vi "Get Fix Type.vi"(8 "error in (no error)":errorcluster, 11 "nmea in":refnum<class "nmea.lvclass">) -> (0 "error out":errorcluster, 2 "Fix Type":T1, 3 "nmea out":refnum<class "nmea.lvclass">)   [LabVIEW 2020, in "nmea.lvlib" / "nmea.lvclass"]
uses:
  nmea.lvclass
  Fix Type.ctl
  nmea.lvclass/nmea.ctl
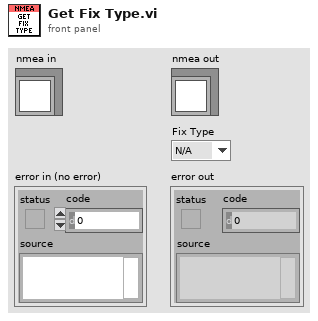
[diagram p1: front panel]
types:
  T1 = typedef "nmea.lvlib/nmea.lvclass/Fix Type.ctl" = enum16{"N/A", "None", "2D", "3D"}
  T2 = typedef "nmea.lvlib/nmea.lvclass/Ref Data.ctl" = cluster{"Latitude":dbl, "Longitude":dbl, "Time":T3, "Status":string, "Speed":dbl, "Course":dbl, "Mag Var":dbl, "Var Dir":string, "Mode":string, "Satellites":T4[], "Next Satellites":T4[], "Active PRNs":i32[], "Fix Type":T1, "DOP":T5, "Fix Mode":T6, "Altitude":dbl, "Geoid":dbl}
  T3 = typedef "LVDateTimeRec.ctl" = cluster{"fractional second":dbl, "second":i32, "minute":i32, "hour":i32, "day of month":i32, "month":i32, "year":i32, "day of week":i32, "day of year":i32, "DST":i32}
  T4 = typedef "nmea.lvlib/nmea.lvclass/Satellite.ctl" = cluster{"PRN":u8, "Channel":u8, "Elevation":u8, "Azimuth":u16, "SNR":u8, "Active":bool}
  T5 = typedef "nmea.lvlib/nmea.lvclass/DOP.ctl" = cluster{"P":dbl, "H":dbl, "V":dbl}
  T6 = typedef "nmea.lvlib/nmea.lvclass/Fix Mode.ctl" = enum16{"Manual", "Auto 2/3D"}
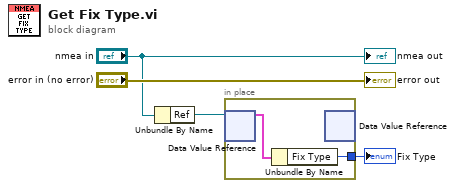
[diagram p0: block diagram]
diagram:
  n1 = Unbundle By Name("nmea in") -> ("Ref"=w3:refnum<data-value>)
  n2 = in-place {
    in-place-border: [w5] -> w1
    n3 = in-place-dvr #1(w3) -> (w6:T2)  [unwired: 1 out]
    n4 = Unbundle By Name(w6) -> ("Fix Type"=w5:T1)
    n5 = in-place-dvr #1() -> ()  [unwired: 1 in, 2 out]
  }
  "Fix Type" <- w1
  "error out" <- "error in (no error)"
  "nmea out" <- "nmea in"
